vi "Generate Last Broadcast Event to View.vi"(0 "Controller Actor in":refnum<class "Controller Actor.lvclass">, 5 "View Enqueuer in":refnum<class "Message Enqueuer.lvclass">, 7 "Event Handler Details":T1, 9 "Event":refnum<class "Event.lvclass">, 11 "error in (no error)":errorcluster) -> (15 "error out":errorcluster)   [LabVIEW 2023, in "Event Actors.lvlib" / "Controller Actor.lvclass"]
uses:
  Controller Actor.lvclass
  Controller Actor.lvclass/Controller Actor.ctl
  Event/Event.lvclass
  Event Handlers/Abstract Event Message for View/Abstract Event Message for View.lvclass
  Event Handler Details.ctl
  <vilib>/ActorFramework/Message Enqueuer/Message Enqueuer.lvclass
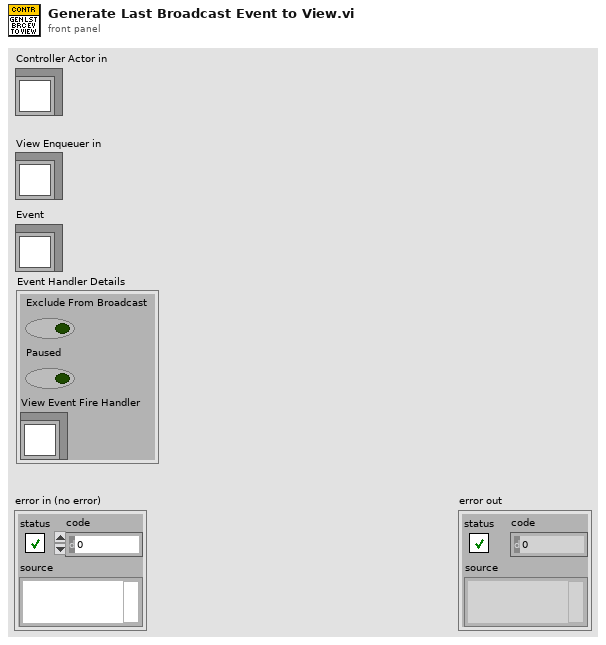
[diagram p1: front panel]
types:
  T1 = typedef "Event Actors.lvlib/Controller Actor.lvclass/Event Handler Details.ctl" = cluster{"Exclude From Broadcast":bool, "Paused":bool, "View Event Fire Handler":refnum<class "Abstract Event Message for View.lvclass">}
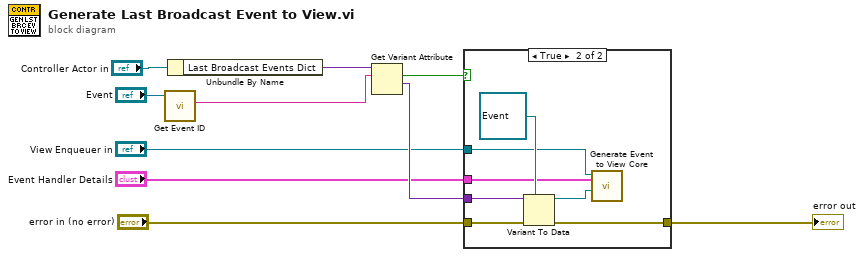
[diagram p0: block diagram]
diagram:
  n1 = call-dynamic "Get Event ID.vi"("Event in"="Event") -> ("Event ID"=w7:string)  [unwired: 8 in, 2 out]
  n2 = Unbundle By Name("Controller Actor in") -> ("Last Broadcast Events Dict"=w10:variant)
  n3 = Get Variant Attribute(Variant=w10, name=w7) -> (found=w4:bool, value=w3:variant)  [unwired: 2 in, 2 out]
  n4 = case shown="True" w4 {
    tunnel: "error in (no error)" -> [w11 w18]
    tunnel: [w11 w17] -> w5
    tunnel: w3 -> [_ w15]
    tunnel: "Event Handler Details" -> [_ w13]
    tunnel: "View Enqueuer in" -> [_ w12]
    frame False {
    }
    frame True {
      n5 = Variant To Data(error in=w18, type=refnum<class "Event.lvclass"> refnum ("Event"), Variant=w15) -> (data=w14:refnum<class "Event.lvclass">, error out=w17:errorcluster)
      n6 = call "Generate Event to View Core.vi"("Event in"=w14, "Event Handler Details"=w13, "Message Enqueuer in"=w12) -> ()  [unwired: 9 in]
    }
  }
  "error out" <- w5
